vi "Z6_Beamline.Calc Northtower State.vi"(0 "i ref in":refnum<vi>, 5 "error in (no error)":errorcluster) -> (14 "i ref out":refnum<vi>, 19 "error out":errorcluster)   [LabVIEW 2014, in "Z6_Beamline.lvlib"]
doc: "This VI calculates the Northtower state of the Z6 Beamline."
uses:
  Z6_Beamline.lvlib
  PH_StatusHandler/PH_StatusHandler.Status.ctl
  PH_Common/PH_Common.lvlib
  PH_StatusHandler/PH_StatusHandler.lvlib
  PH_BL-Master/PH_BL-Master.lvlib
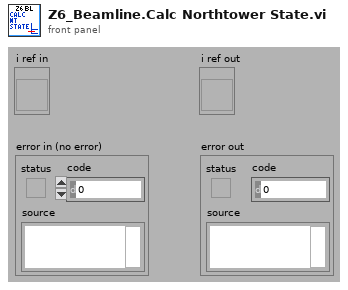
[diagram p1: front panel]
types:
  T1 = typedef "PH_StatusHandler.lvlib/PH_StatusHandler.Status.ctl" = i16
  T2 = typedef "Z6_Beamline.lvlib/Z6_Beamline.i attribute.ctl" = cluster{"Subs ok GUI Refs":T3, "Refs BL Northtower":refnum<vi>[], "Refs BL Southtower":refnum<vi>[], "Refs BL 100TW COS":refnum<vi>[], "State Subsystems":cluster{"Northtower":bool, "Southtower":bool, "Frontends":bool, "100TW COS":bool}, "Z6 Beamline Status Subscriber Information":T4, "Color State PHELIX":i16}
  T3 = typedef "Z6_Beamline.lvlib/Z6_Beamline.Subsystem ok GUI Refs.ctl" = cluster{"Northtower ok":refnum<vi>, "Southtower ok":refnum<vi>, "Frontends ok":refnum<vi>, "100TW COS ok":refnum<vi>}
  T4 = typedef "Z6_Beamline.lvlib/Z6_Beamline.Status Subscriber Information.ctl" = cluster{"BL Z6 Shutter":T5, "CH 10":T5, "CH 11":T5, "ST Flip Cam":T5, "ST Flip DB":T5, "BL Z6 Dump":T5}
  T5 = typedef "PH_BL-Master.lvlib/PH_BL-Master.Status Subscriber Information.ctl" = cluster{"Index of element":i32, "Attributeset":T6}
  T6 = typedef "PH_BL-Master.lvlib/PH_BL-Master.Attribute Set.ctl" = enum16{"Boolean Status Service Subscriber", "Picture Status Service Subscriber"}
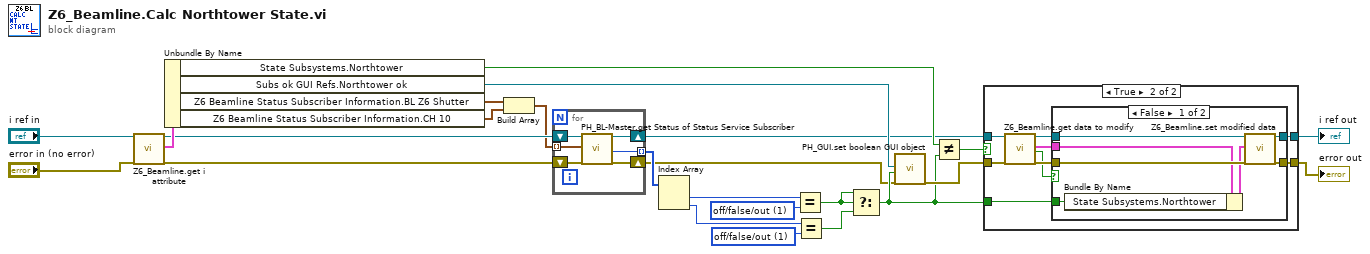
[diagram p0: block diagram]
diagram:
  w13 = T1 1 items=["no info", "off/false/out", "on/true/in", "Failure", "Alarm", "Status 1", "Status 2", "Status 3"] ("element")
  w15 = T1 1 items=["no info", "off/false/out", "on/true/in", "Failure", "Alarm", "Status 1", "Status 2", "Status 3"] ("element")
  n1 = call "Z6_Beamline.get i attribute.vi"("i ref in"="i ref in", "error in (no error)"="error in (no error)") -> ("i ref out"=w7:refnum<vi>, "i attribute"=w24:T2, "error out"=w6:errorcluster)  [unwired: 15 in]
  n2 = Unbundle By Name(w24) -> ("State Subsystems.Northtower"=w21:bool, "Subs ok GUI Refs.Northtower ok"=w23:refnum<vi>, "Z6 Beamline Status Subscriber Information.BL Z6 Shutter"=w3:T5, "Z6 Beamline Status Subscriber Information.CH 10"=w2:T5)
  n3 = Build Array(w3, w2) -> (w1:T5[])
  n4 = for {
    tunnel: w1 -> [w26] mode=indexing
    shift-right: [w29] -> w4
    shift-left: w6 -> [w30]
    shift-right: [w27] -> w5
    shift-left: w7 -> [w28]
    tunnel: [w25] -> w17 mode=indexing
    n5 = call "PH_BL-Master.get Status of Status Service Subscriber.vi"("i ref in"=w28, "Wanted Status Subscriber Information"=w26, "error in (no error)"=w30) -> ("i ref out"=w27:refnum<vi>, "Status"=w25:T1, "error out"=w29:errorcluster)  [unwired: 11 in, 3 out]
  }
  n6 = Index Array(array=w17) -> (element #1=w16:T1, element #2=w11:T1)  [unwired: 2 in]
  n7 = Equal?(x=w16, y=w15) -> (x = y?=w12:bool)
  n8 = Equal?(x=w11, y=w13) -> (x = y?=w10:bool)
  n9 = Select(t=w12, s=w12, f=w10) -> (s? t:f=w14:bool)
  n10 = call "PH_GUI.set boolean GUI object.vi"("Boolean Knob GUI Ref"=w23, "Value"=w14, "error in (no error)"=w4) -> ("error out"=w20:errorcluster)  [unwired: 16 in]
  n11 = Not Equal?(x=w21, y=w14) -> (x != y?=w22:bool)
  n12 = case shown="True" w22 {
    tunnel: w5 -> [w32 w37]
    tunnel: [w32 w36] -> w18
    tunnel: w20 -> [w31 w35]
    tunnel: [w31 w34] -> w19
    tunnel: w14 -> [_ w33]
    frame False {
    }
    frame True {
      n13 = call "Z6_Beamline.get data to modify.vi"("i ref in"=w37, "error in (no error)"=w35) -> ("i ref out"=w40:refnum<vi>, "i attribute"=w38:T2, "timed out"=w39:bool, "error out"=w41:errorcluster)  [unwired: 14 in]
      n14 = case shown="False" w39 {
        tunnel: w41 -> [w48 w49]
        tunnel: w40 -> [w47 w50]
        tunnel: [w46 w49] -> w34
        tunnel: [w45 w50] -> w36
        tunnel: w38 -> [w44 _]
        tunnel: w33 -> [w42 _]
        frame False {
          n15 = Bundle By Name(cluster=w44, "State Subsystems.Northtower"=w42) -> (w43:T2)
          n16 = call "Z6_Beamline.set modified data.vi"("i ref in"=w47, "i attribute"=w43, "error in (no error)"=w48) -> ("i ref out"=w45:refnum<vi>, "error out"=w46:errorcluster)  [unwired: 15 in]
        }
        frame True {
        }
      }
    }
  }
  "i ref out" <- w18
  "error out" <- w19
